vi "Add Event.vi"(8 "error in (no error)":errorcluster, 9 "Controller Event Handler":refnum<class "Abstract Event Handler for Controller.lvclass">, 10 "Event":refnum<class "Event.lvclass">, 11 "Controller in":refnum<class "Controller.lvclass">) -> (0 "error out":errorcluster, 3 "Controller out":refnum<class "Controller.lvclass">)   [LabVIEW 2023, in "MVC Actors.lvlib" / "Controller.lvclass"]
doc: "This method adds an event to the list of the events handled by the Controller Actor. If the Controller Actor wants to handle the events from the View, a concrete implementation of the <b>\"Abstract Event Handler for Controller.lvclass\"</b> should be wired to the <b>\"Controller Event Handler\"</b> terminal."
uses:
  Controller.lvclass
  Controller.lvclass/Controller.ctl
  <vilib>/ErrorRing/Error Ring.xnode
  <vilib>/Utility/error.llb/Error Cluster From Error Code.vi
  Event/Event.lvclass
  Event Handlers/Abstract Event Handler for Controller/Abstract Event Handler for Controller.lvclass
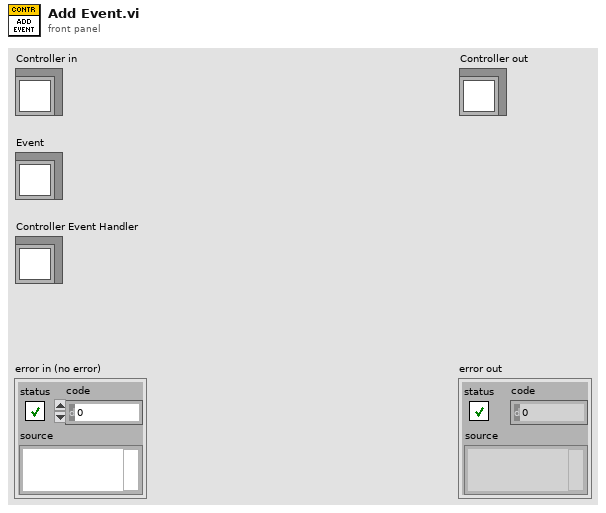
[diagram p1: front panel]
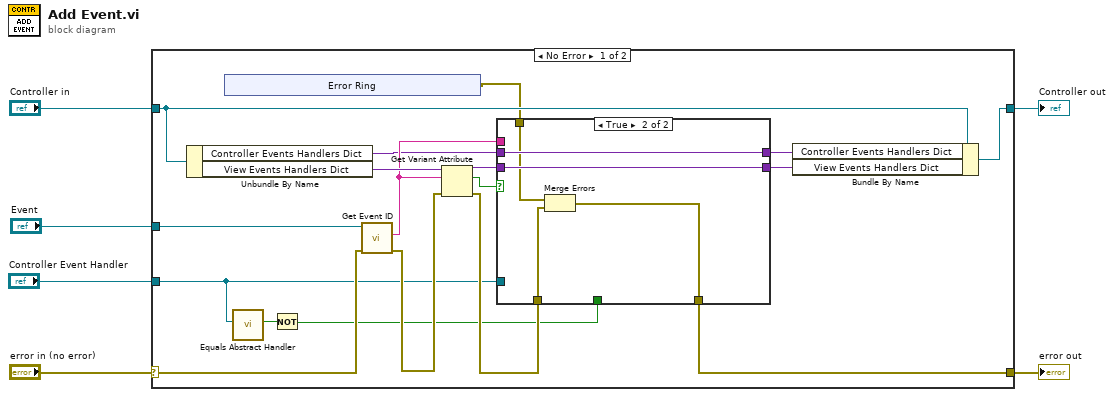
[diagram p0: block diagram]
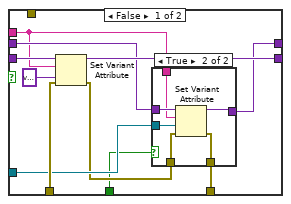
[diagram p2: hidden frame]
diagram:
  n1 = case shown="No Error" "error in (no error)" {
    selector: "error in (no error)" -> [w22 w54]
    tunnel: [w12 w54] -> w5
    tunnel: [w15 w53] -> w3
    tunnel: "Controller in" -> [w24 w53]
    tunnel: "Event" -> [w23 _]
    tunnel: "Controller Event Handler" -> [w10 _]
    frame No Error {
      n2 = Unbundle By Name(w24) -> ("Controller Events Handlers Dict"=w13:variant, "View Events Handlers Dict"=w21:variant)
      n3 = xnode "Error Ring"() -> ("error out"=w7:errorcluster)
      n4 = call "Equals Abstract Handler.vi"("Controller Event Fire Handler"=w10) -> ("Is Abstract Event Handler"=w9:bool)  [unwired: 10 in]
      n5 = Not(x=w9) -> (.not. x?=w8:bool)
      n6 = call-dynamic "Get Event ID.vi"("error in (no error)"=w22, "Event in"=w23) -> ("error out"=w20:errorcluster, "Event ID"=w17:string)  [unwired: 7 in, 1 out]
      n7 = Get Variant Attribute(Variant=w21, name=w17, error in=w20) -> (duplicate Variant=w18:variant, found=w19:bool, error out=w16:errorcluster)  [unwired: 1 in, 1 out]
      n8 = case shown="True" w19 {
        tunnel: w18 -> [w39 w52]
        tunnel: w17 -> [w34 _]
        tunnel: w16 -> [w38 w49]
        tunnel: w7 -> [_ w48]
        tunnel: [w36 w52] -> w14
        tunnel: w13 -> [w35 w50]
        tunnel: w10 -> [w33 _]
        tunnel: [w31 w51] -> w12
        tunnel: w8 -> [w30 _]
        tunnel: [w29 w50] -> w11
        frame False {
          n9 = Set Variant Attribute(Variant=w39, name=w34, value=variant ("Events Dict"), error in=w38) -> (Variant out=w36:variant, error out=w32:errorcluster)  [unwired: 1 out]
          n10 = case shown="True" w30 {
            tunnel: w35 -> [w40 w47]
            tunnel: w34 -> [_ w46]
            tunnel: w33 -> [_ w45]
            tunnel: w32 -> [w41 w44]
            tunnel: [w41 w43] -> w31
            tunnel: [w40 w42] -> w29
            frame False {
            }
            frame True {
              n11 = Set Variant Attribute(Variant=w47, name=w46, value=w45, error in=w44) -> (Variant out=w42:variant, error out=w43:errorcluster)  [unwired: 1 out]
            }
          }
        }
        frame True {
          n12 = Merge Errors(w48, w49) -> (w51:errorcluster)
        }
      }
      n13 = Bundle By Name(cluster=w24, "Controller Events Handlers Dict"=w11, "View Events Handlers Dict"=w14) -> (w15:refnum<class "Controller.lvclass">)
    }
    frame Error {
    }
  }
  "error out" <- w5
  "Controller out" <- w3
